vi "Initialize.vi"(8 "error in":errorcluster, 10 "parameters":variant, 11 "cRIO in":refnum<class "cRIO  node root.lvclass">) -> (0 "error out":errorcluster, 2 "summary":T2[](array[typedef]), 3 "data value reference":T1)   [LabVIEW 2014, in "cRIO  node root.lvclass"]
doc: "This Vi initializes the data of a node its default state.\nThe object is not created inside of this ViI, beacuase it is created from a File depending on user selection."
uses:
  cRIO  node root.lvclass
  <vilib>/NI/Configuration Framework/Node/Summary.ctl
  <vilib>/NI/Configuration Framework/Node/NodeRef.ctl
  <vilib>/NI/Configuration Framework/Node/NISE_CEF_Node.lvclass
  cRIO configuration/cRIO configuration.lvclass
  cRIO  node root.lvclass/cRIO  node root.ctl
  <vilib>/NI/Configuration Framework/serializable configuration/set metadata property.vi
  <vilib>/NI/Configuration Framework/serializable node/NISE_CEF_serializable node.lvclass
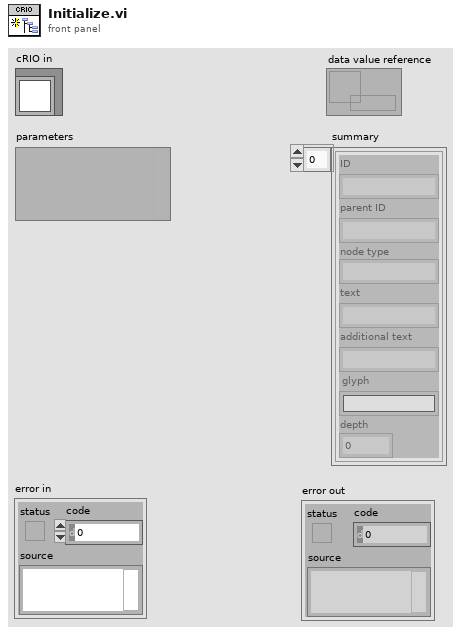
[diagram p1: front panel]
types:
  T1 = typedef "NISE_CEF_Node.lvclass/NodeRef.ctl" = refnum<data-value>
  T2 = typedef "NISE_CEF_Node.lvclass/Summary.ctl" = cluster{"ID":string, "parent ID":string, "node type":string, "text":string, "additional text":string, "glyph":string, "depth":i32}
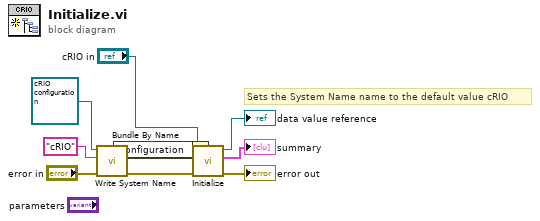
[diagram p0: block diagram]
diagram:
  # "Sets the System Name name to the default value cRIO"
  n1 = call "Write System Name.vi"("error in (no error)"="error in", "System Name"="cRIO", "crio configuration in"=refnum<class "cRIO configuration.lvclass"> refnum ("crio configuration.lvclass")) -> ("error out"=w2:errorcluster, "crio configuration out"=w3:refnum<class "cRIO configuration.lvclass">)  [unwired: 7 in]
  n2 = Bundle By Name(cluster="cRIO in", "configuration"=w3) -> (w7:refnum<class "cRIO  node root.lvclass">)
  n3 = call-parent "Initialize.vi"("error in"=w2, "node in"=w7) -> ("error out"=→"error out":errorcluster, "summary"=→"summary":T2[], "data value reference"=→"data value reference":T1)  [unwired: 7 in]
